vi "GetArray.vi"() -> ()   [LabVIEW 2020]
uses:
  859b58b0-79df-43f2-a2e9-99a1650faf3a.vi
panel:
  out "Waveform Chart":T1(graph)
  in  "stop":bool
  in  "format string":string
  out "Table Control 2":string[][](table)
  in  "expected output size  (4096)":u32
  in  "working directory":path=path ""
  out "standard output":string
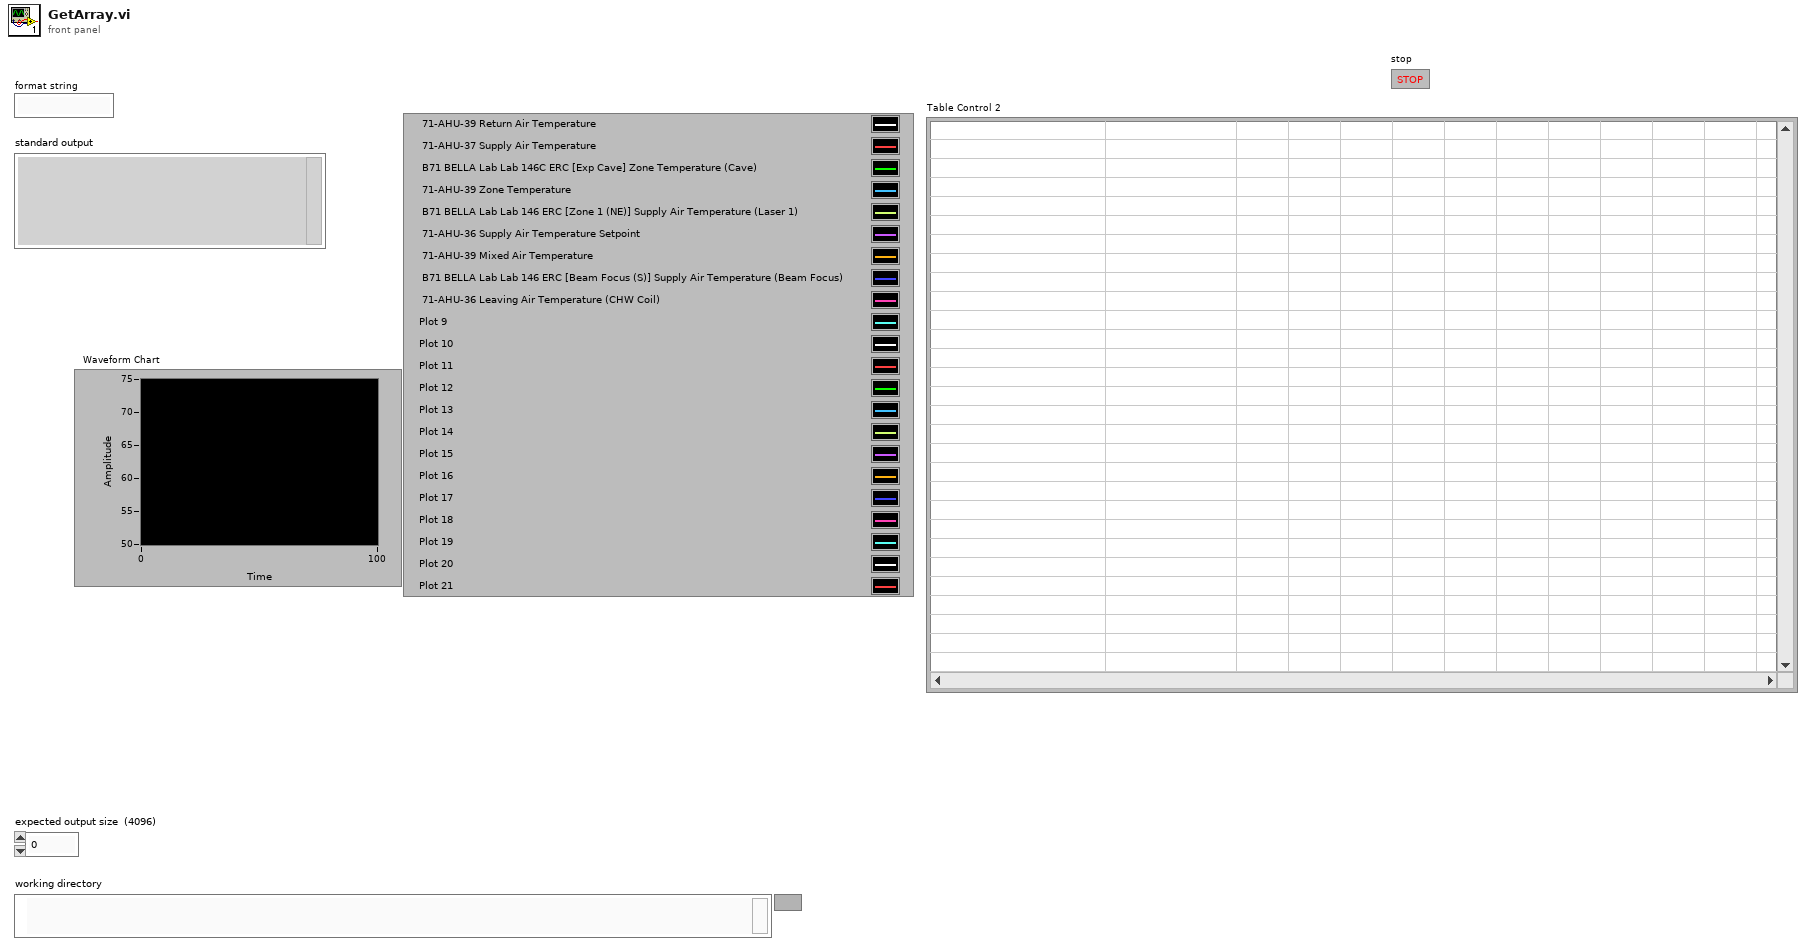
[diagram p1: front panel]
types:
  T1 = cluster{"[0]":dbl, "[1]":dbl, "[2]":dbl, "[3]":dbl, "[4]":dbl, "[5]":dbl, "[6]":dbl, "[7]":dbl, "[8]":dbl}
  T2 = cluster{"[0]":string, "[1]":string, "[2]":string, "[3]":string, "[4]":string, "[5]":string, "[6]":string, "[7]":string, "[8]":string}
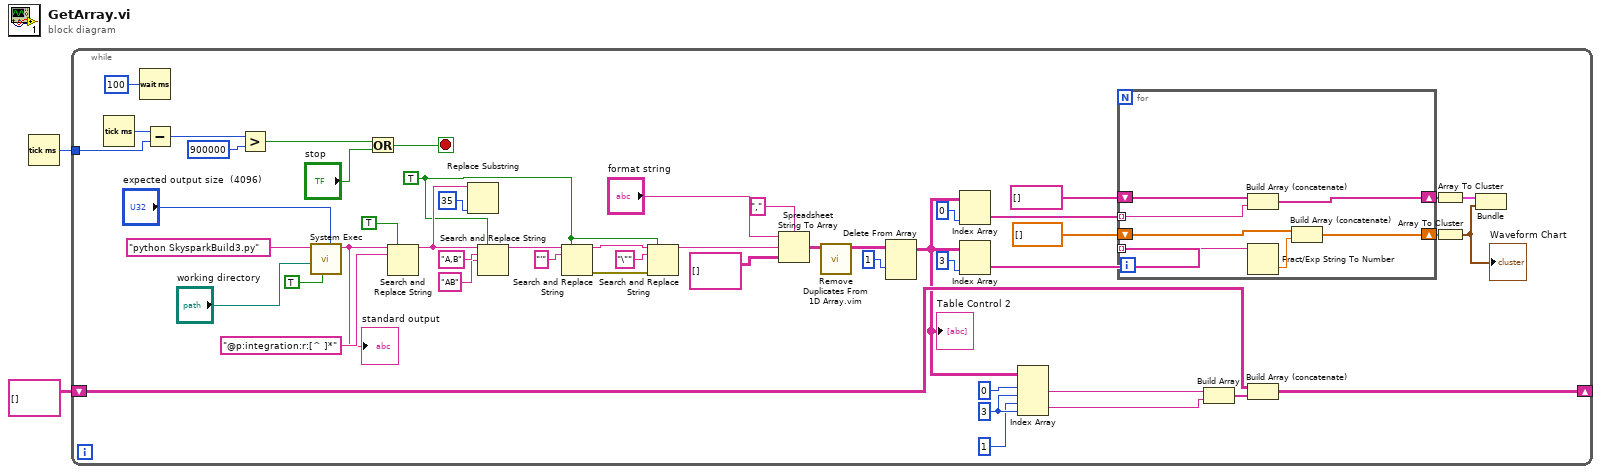
[diagram p0: block diagram]
diagram:
  n1 = Tick Count (ms)() -> (millisecond timer value=w1:u32)
  n2 = while {
    shift-right: [w29] -> _
    shift-left: string[][] [] -> [w44]
    tunnel: w1 -> [w47]
    stop <- w18 stop-if-true
    w28 = 3 ("disabled index (col)")
    w5 = TRUE ("replace all? (F)")
    n3 = Tick Count (ms)() -> (millisecond timer value=w48:u32)
    n4 = Wait (ms)(milliseconds to wait=u32 100) -> ()  [unwired: 1 out]
    n5 = Subtract(x=w48, y=w47) -> (x-y=w46:u32)
    n6 = Greater?(x=w46, y=u32 900000) -> (0:w20:bool)
    n7 = call <vilib>:"System Exec.vi"("expected output size  (4096)"="expected output size  (4096)", "run minimized? (F)"=TRUE, "working directory"="working directory", "command line"="python SkysparkBuild3.py") -> ("standard output"=w31:string)  [unwired: 4 in, 3 out]
    "standard output" <- w31
    n8 = Or(x=w20, y="stop") -> (x .or. y?=w18:bool)
    n9 = Search and Replace String(replace all?=TRUE ("replace all? (F)"), input string=w31, search string="@p:integration:r:[^ ]*") -> (result string=w32:string)  [unwired: 5 in, 3 out]
    n10 = Replace Substring(2:35 ("length (len. of substring)"), 5:w32) -> ()  [unwired: 2 in, 2 out]
    n11 = Search and Replace String(replace all?=w5, input string=w32, search string="A,B" ("substring (\"\")"), replace string="AB" ("replace string (\"\")")) -> (result string=w9:string)  [unwired: 4 in, 3 out]
    n12 = Search and Replace String(replace all?=w5, input string=w9, search string="'") -> (result string=w8:string, error out=w7:errorcluster)  [unwired: 5 in, 2 out]
    n13 = Search and Replace String(replace all?=w5, input string=w8, search string="\"", error in=w7) -> (result string=w6:string)  [unwired: 4 in, 3 out]
    n14 = Spreadsheet String To Array(delimiter (Tab)=",", format string="format string", spreadsheet string=w6, array type (2D Dbl)=string[][] []) -> (array=w40:string[][])
    n15 = call "Remove Duplicates From 1D Array.vim"("array"=w40) -> ("array with duplicates removed"=w39:string[][])  [unwired: 10 in]
    n16 = Delete From Array(array=w39, index (row)=1) -> (array with subset deleted=w17:string[][])  [unwired: 2 in, 1 out]
    "Table Control 2" <- w17
    n17 = Index Array(array=w17, index (col)=0 ("disabled index (col)")) -> (element=w16:string[])  [unwired: 1 in]
    n18 = Index Array(array=w17, index (col)=3 ("disabled index (col)")) -> (element=w22:string[])  [unwired: 1 in]
    n19 = Index Array(array=w17, index (row) #1=0 ("index (row)"), index (col) #1=w28, index (row) #2=1 ("disabled index (row)"), index (col) #2=w28) -> (element #1=w25:string, element #2=w26:string)
    n20 = for {
      tunnel: w22 -> [w60] mode=indexing
      shift-right: [w58] -> w13
      shift-left: dbl[] [] -> [w57]
      tunnel: w16 -> [w54] mode=indexing
      shift-right: [w56] -> w12
      shift-left: string[] [] -> [w55]
      n21 = Build Array (concatenate)(w55, w54) -> (w56:string[])
      n22 = Fract/Exp String To Number(string=w60) -> (number=w59:dbl)  [unwired: 3 in, 1 out]
      n23 = Build Array (concatenate)(w57, w59) -> (w58:dbl[])
    }
    n24 = Build Array(w25, w26) -> (w24:string[])
    n25 = Build Array (concatenate)(w44, w24) -> (w29:string[][])
    n26 = Array To Cluster(array=w12) -> (cluster=w11:T2)
    n27 = Array To Cluster(array=w13) -> (cluster=w10:T1)
    "Waveform Chart" <- w10
    n28 = Bundle(w11, w10) -> ()  [unwired: 1 in, 1 out]
  }
